vi "左工位判定.vi"(7 "Result":refnum<vi>, 10 "左工位判定":T1, 11 "XY曲线":cluster{"X":dbl[], "Y":dbl[]}[](array[cluster])) -> (2 "大小":i32, 3 "OK？":bool)   [LabVIEW 2020]
uses:
  Global_Variable/Global.vi
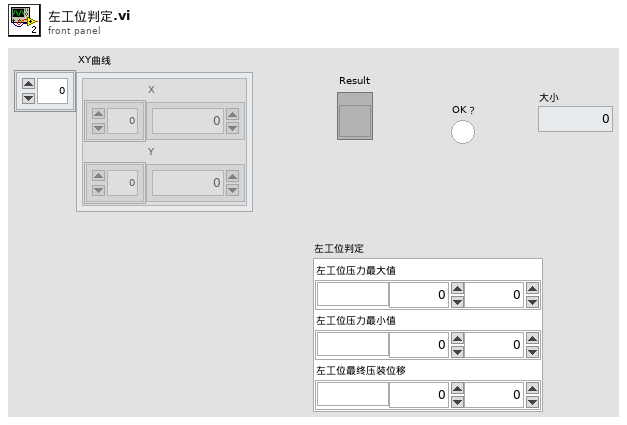
[diagram p1: front panel]
types:
  T1 = cluster{"左工位压力最大值":cluster{"单位":string, "下限":dbl, "上限":dbl}, "左工位压力最小值":cluster{"单位":string, "下限":dbl, "上限":dbl}, "左工位最终压装位移":cluster{"单位":string, "下限":dbl, "上限":dbl}}
  T2 = cluster{"X ":cluster{"单位":string, "下限":dbl, "上限":dbl}, "Y":cluster{"单位":string, "下限":dbl, "上限":dbl}}
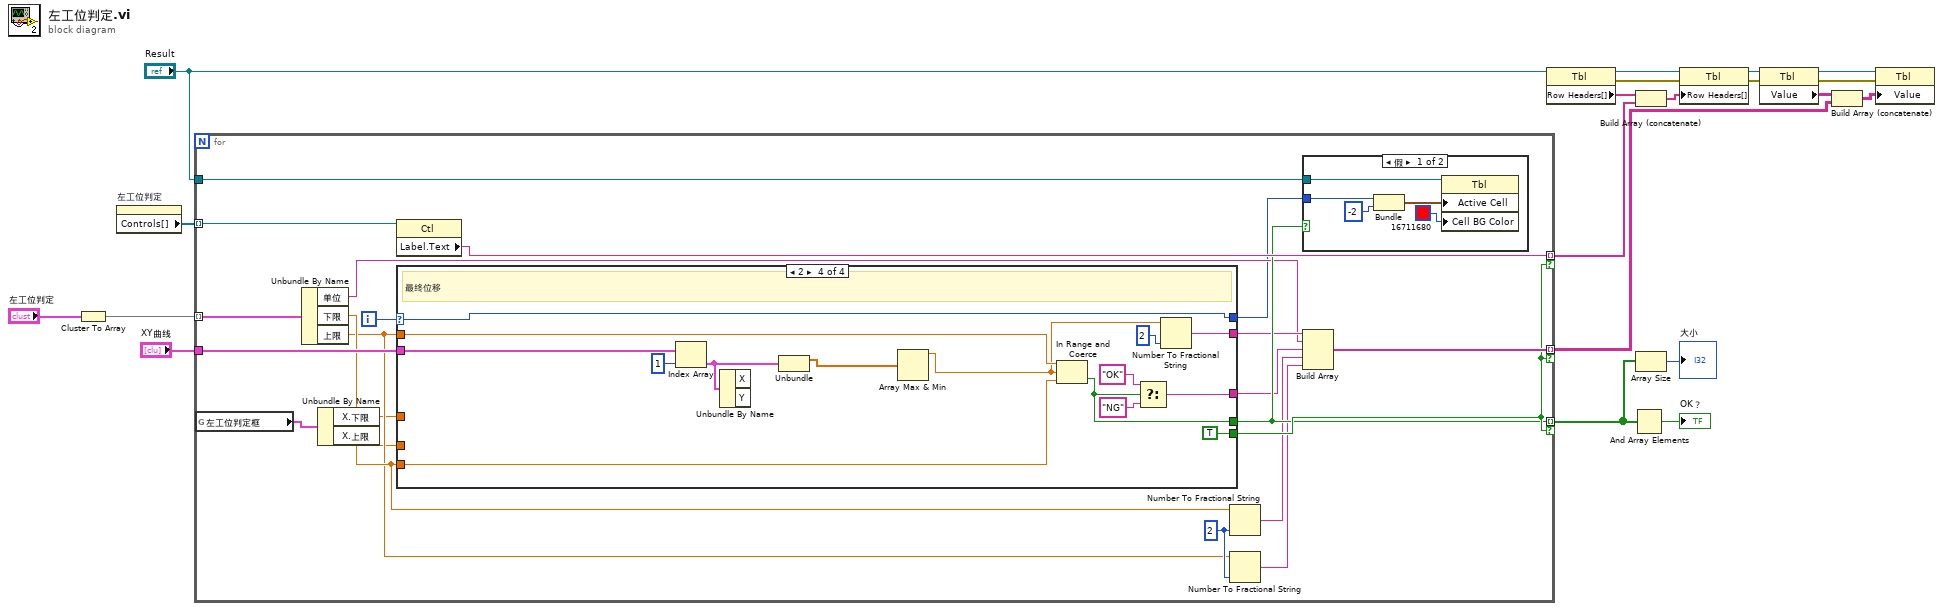
[diagram p0: block diagram]
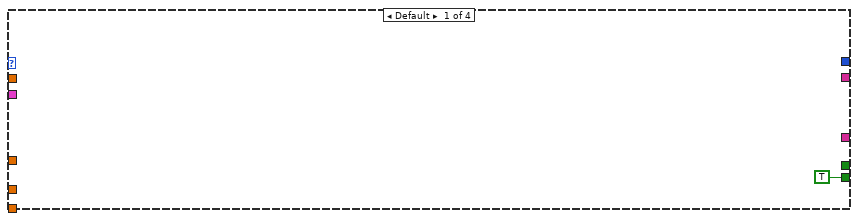
[diagram p3: hidden frame]
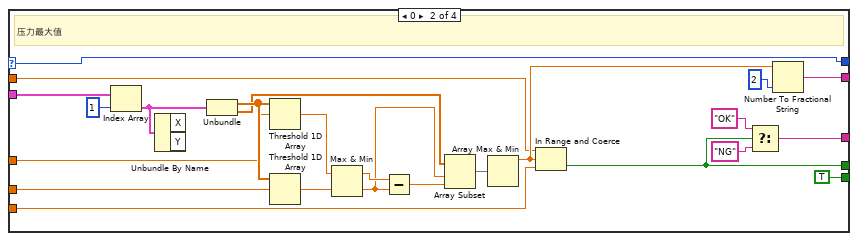
[diagram p4: hidden frame]
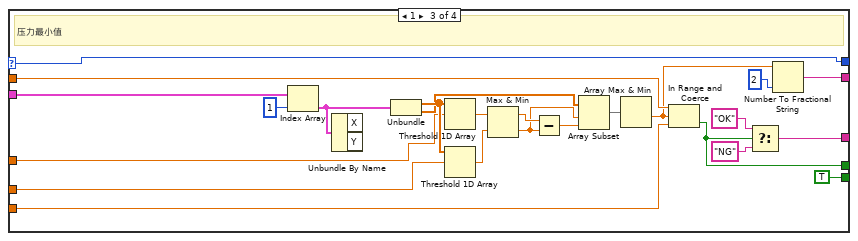
[diagram p5: hidden frame]
diagram:
  n1 = Cluster To Array(cluster="左工位判定") -> (array=w20:cluster{"单位":string, "下限":dbl, "上限":dbl}[])
  n2 = property on="左工位判定" class="Clust (严格)"() -> ("Controls[]"=w1:refnum<vi>[])  [unwired: 2 in, 2 out]
  n3 = for {
    tunnel: w20 -> [w41] mode=indexing
    tunnel: w1 -> [w39] mode=indexing
    tunnel: "XY曲线" -> [w38]
    tunnel: [w30] -> w3 mode=indexing if=w31
    tunnel: [w34] -> w7 mode=indexing if=w31
    tunnel: [w33] -> w9 mode=indexing if=w31
    tunnel: "Result" -> [w32]
    i -> [w40]
    w37 = i16 2 ("精度(6)")
    n4 = global read "Global.vi" "左工位判定框"() -> (w21:T2)
    n5 = Unbundle By Name(w41) -> ("单位"=w28:string, "下限"=w36:dbl, "上限"=w35:dbl)
    n6 = Unbundle By Name(w21) -> ("X.下限"=w23:dbl, "X.上限"=w22:dbl)
    n7 = property class="Ctl"(reference=w39) -> ("Label.Text"=w33:string)  [unwired: 1 in, 2 out]
    n8 = case shown="2" w40 {
      selector: w40 -> [_ w52 w77 w100]
      tunnel: w38 -> [_ w71 w95 w110]
      tunnel: [_ w68 w92 w107] -> w27
      tunnel: [_ w67 w91 w106] -> w30
      tunnel: w36 -> [_ w51 w76 w99]
      tunnel: w35 -> [_ w50 w75 w98]
      tunnel: [TRUE TRUE TRUE TRUE] -> w31
      tunnel: [_ w53 w78 w101] -> w29
      tunnel: [_ w52 w77 w100] -> w24
      tunnel: w23 -> [_ w49 w73 _]
      tunnel: w22 -> [_ w48 w72 _]
      frame Default {
      }
      frame 0 {
        # "压力最大值"
        n9 = Index Array(array=w71, index=1 ("索引")) -> (element=w62:cluster{"X":dbl[], "Y":dbl[]})
        n10 = Unbundle By Name(w62) -> ()  [unwired: 2 out]
        n11 = Unbundle(w62) -> ("X"=w61:dbl[], "Y"=w58:dbl[])
        n12 = Threshold 1D Array(2:w49, 3:w61) -> (0:w65:dbl)  [unwired: 1 in]
        n13 = Threshold 1D Array(2:w48, 3:w61) -> (0:w64:dbl)  [unwired: 1 in]
        n14 = Max & Min(x=w65, y=w64) -> (max(x,y)=w63:dbl, min(x,y)=w59:dbl)
        n15 = Subtract(x=w63, y=w59) -> (x-y=w60:dbl)
        n16 = Array Subset(array=w58, index=w59, length=w60) -> (w57:dbl[])
        n17 = Array Max & Min(array=w57) -> (max value=w54:dbl)  [unwired: 3 out]
        n18 = In Range and Coerce(upper limit=w50, x=w54, lower limit=w51) -> (In Range?=w67:bool)  [unwired: 1 out]
        n19 = Select(t="OK", s=w67, f="NG") -> (s? t:f=w68:string)
        n20 = Number To Fractional String(number=w54, precision (6)=i16 2 ("精度(6)")) -> (F-format string=w53:string)  [unwired: 2 in]
      }
      frame 1 {
        # "压力最小值"
        n21 = Index Array(array=w95, index=1 ("索引")) -> (element=w86:cluster{"X":dbl[], "Y":dbl[]})
        n22 = Unbundle By Name(w86) -> ()  [unwired: 2 out]
        n23 = Unbundle(w86) -> ("X"=w85:dbl[], "Y"=w82:dbl[])
        n24 = Threshold 1D Array(2:w73, 3:w85) -> (0:w89:dbl)  [unwired: 1 in]
        n25 = Threshold 1D Array(2:w72, 3:w85) -> (0:w88:dbl)  [unwired: 1 in]
        n26 = Max & Min(x=w89, y=w88) -> (max(x,y)=w87:dbl, min(x,y)=w83:dbl)
        n27 = Subtract(x=w87, y=w83) -> (x-y=w84:dbl)
        n28 = Array Subset(array=w82, index=w83, length=w84) -> (w81:dbl[])
        n29 = Array Max & Min(array=w81) -> (min value=w74:dbl)  [unwired: 3 out]
        n30 = In Range and Coerce(upper limit=w75, x=w74, lower limit=w76) -> (In Range?=w91:bool)  [unwired: 1 out]
        n31 = Select(t="OK", s=w91, f="NG") -> (s? t:f=w92:string)
        n32 = Number To Fractional String(number=w74, precision (6)=i16 2 ("精度(6)")) -> (F-format string=w78:string)  [unwired: 2 in]
      }
      frame 2 {
        # "最终位移"
        n33 = Index Array(array=w110, index=1 ("索引")) -> (element=w104:cluster{"X":dbl[], "Y":dbl[]})
        n34 = Unbundle By Name(w104) -> ()  [unwired: 2 out]
        n35 = Unbundle(w104) -> ("X"=w97:dbl[])  [unwired: 1 out]
        n36 = Array Max & Min(array=w97) -> (max value=w96:dbl)  [unwired: 3 out]
        n37 = In Range and Coerce(upper limit=w98, x=w96, lower limit=w99) -> (In Range?=w106:bool)  [unwired: 1 out]
        n38 = Select(t="OK", s=w106, f="NG") -> (s? t:f=w107:string)
        n39 = Number To Fractional String(number=w96, precision (6)=i16 2 ("精度(6)")) -> (F-format string=w101:string)  [unwired: 2 in]
      }
    }
    n40 = Number To Fractional String(number=w36, precision (6)=w37) -> (F-format string=w26:string)  [unwired: 2 in]
    n41 = Number To Fractional String(number=w35, precision (6)=w37) -> (F-format string=w25:string)  [unwired: 2 in]
    n42 = case shown="假" w30 {
      tunnel: w32 -> [w46 _]
      tunnel: w24 -> [w42 _]
      frame False {
        n43 = Bundle(w42, -2) -> (w44:cluster{i32, i32})  [unwired: 1 in]
        n44 = property class="Tbl"(reference=w46, "Active Cell"=w44, "Cell BG Color"=u32 16711680 ("活动单元格:单元格背景色")) -> ()  [unwired: 1 in, 2 out]
      }
      frame True {
      }
    }
    n45 = Build Array(w29, w28, w27, w26, w25) -> (w34:string[])
  }
  n46 = property class="Tbl"(reference="Result") -> (reference out=w11:refnum<vi>, error out=w16:errorcluster, "Row Headers[]"=w8:string[])  [unwired: 1 in]
  n47 = And Array Elements(Boolean array=w3) -> (logical AND=→"OK？":bool)
  n48 = Build Array (concatenate)(w8, w9) -> (w10:string[])
  n49 = Array Size(array=w3) -> (size(s)=→"大小":i32)
  n50 = property class="Tbl"(reference=w11, error in=w16, "Row Headers[]"=w10) -> (reference out=w12:refnum<vi>, error out=w15:errorcluster)
  n51 = property class="Tbl"(reference=w12, error in=w15) -> (reference out=w13:refnum<vi>, error out=w14:errorcluster, "Value"=w17:string[][])
  n52 = Build Array (concatenate)(w17, w7) -> (w18:string[][])
  n53 = property class="Tbl"(reference=w13, error in=w14, "Value"=w18) -> ()  [unwired: 2 out]
